vi "Set Refnums.vi"   [LabVIEW 2012]
uses:
  <vilib>/Rock Robotics/WPI/DriverStation/WPI_DriverStationRobotMode2.ctl
  Global Refnums.vi
  Robot Global Data.vi
  Global Variables.vi
types:
  T1 = typedef "WPI_DriverStationRobotMode2.ctl" = enum16{"Autonomous Disabled", "Autonomous Enabled", "Teleop Disabled", "Teleop Enabled", "Timeout", "Finish", "Test Disabled", "Test Enabled"}
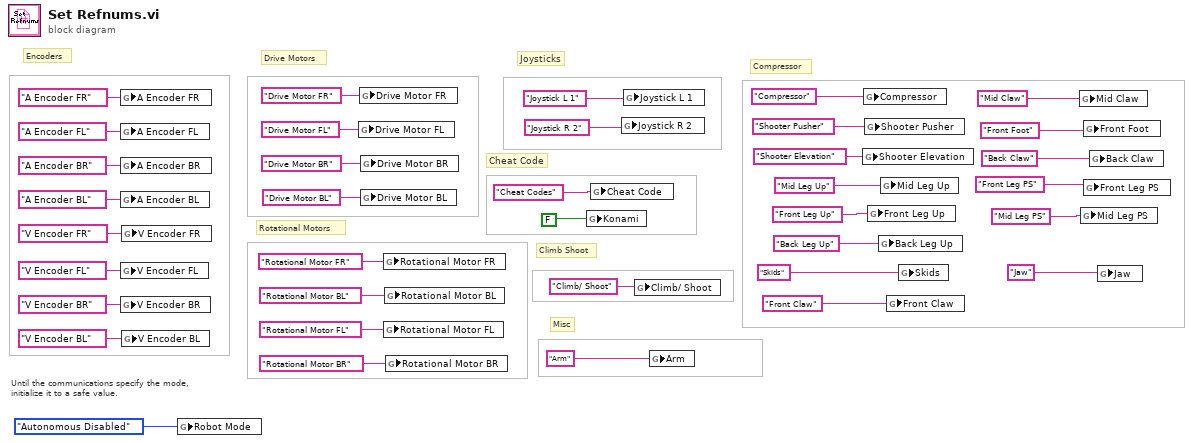
[diagram p0: block diagram]
diagram:
  # "Misc"
  # "Climb Shoot"
  # "Cheat Code"
  # "Until the communications specify the mode,\ninitialize it to a safe value."
  # "Compressor"
  # "Joysticks"
  # "Rotational Motors"
  # "Encoders"
  # "Drive Motors"
  n1 = global write "Global Refnums.vi" "A Encoder FR"("A Encoder FR") -> ()
  n2 = global write "Global Refnums.vi" "A Encoder FL"("A Encoder FL") -> ()
  n3 = global write "Global Refnums.vi" "A Encoder BR"("A Encoder BR") -> ()
  n4 = global write "Global Refnums.vi" "A Encoder BL"("A Encoder BL") -> ()
  n5 = global write "Global Refnums.vi" "V Encoder FL"("V Encoder FL") -> ()
  n6 = global write "Global Refnums.vi" "V Encoder BR"("V Encoder BR") -> ()
  n7 = global write "Global Refnums.vi" "V Encoder FR"("V Encoder FR") -> ()
  n8 = global write "Global Refnums.vi" "V Encoder BL"("V Encoder BL") -> ()
  n9 = global write "Robot Global Data.vi" "Robot Mode"(WPI_DriverStationRobotMode2."Autonomous Disabled" ("Robot Mode")) -> ()
  n10 = global write "Global Refnums.vi" "Drive Motor FL"("Drive Motor FL") -> ()
  n11 = global write "Global Refnums.vi" "Drive Motor FR"("Drive Motor FR") -> ()
  n12 = global write "Global Refnums.vi" "Drive Motor BR"("Drive Motor BR") -> ()
  n13 = global write "Global Refnums.vi" "Drive Motor BL"("Drive Motor BL") -> ()
  n14 = global write "Global Refnums.vi" "Rotational Motor FR"("Rotational Motor FR") -> ()
  n15 = global write "Global Refnums.vi" "Rotational Motor FL"("Rotational Motor FL") -> ()
  n16 = global write "Global Refnums.vi" "Rotational Motor BL"("Rotational Motor BL") -> ()
  n17 = global write "Global Refnums.vi" "Rotational Motor BR"("Rotational Motor BR") -> ()
  n18 = global write "Global Variables.vi" "Konami"(FALSE) -> ()
  n19 = global write "Global Refnums.vi" "Cheat Code"("Cheat Codes" ("refnum name")) -> ()
  n20 = global write "Global Refnums.vi" "Joystick R 2"("Joystick R 2") -> ()
  n21 = global write "Global Refnums.vi" "Joystick L 1"("Joystick L 1") -> ()
  n22 = global write "Global Refnums.vi" "Climb/ Shoot"("Climb/ Shoot") -> ()
  n23 = global write "Global Refnums.vi" "Arm"("Arm" ("Arm")) -> ()
  n24 = global write "Global Refnums.vi" "Shooter Elevation"("Shooter Elevation" ("refnum name")) -> ()
  n25 = global write "Global Refnums.vi" "Compressor"("Compressor" ("refnum name")) -> ()
  n26 = global write "Global Refnums.vi" "Shooter Pusher"("Shooter Pusher" ("refnum name")) -> ()
  n27 = global write "Global Refnums.vi" "Front Leg Up"("Front Leg Up" ("refnum name")) -> ()
  n28 = global write "Global Refnums.vi" "Back Leg Up"("Back Leg Up" ("refnum name")) -> ()
  n29 = global write "Global Refnums.vi" "Mid Leg Up"("Mid Leg Up" ("refnum name")) -> ()
  n30 = global write "Global Refnums.vi" "Front Claw"("Front Claw" ("refnum name")) -> ()
  n31 = global write "Global Refnums.vi" "Skids"("Skids" ("refnum name")) -> ()
  n32 = global write "Global Refnums.vi" "Mid Claw"("Mid Claw" ("refnum name")) -> ()
  n33 = global write "Global Refnums.vi" "Mid Leg PS"("Mid Leg PS" ("refnum name")) -> ()
  n34 = global write "Global Refnums.vi" "Front Foot"("Front Foot" ("refnum name")) -> ()
  n35 = global write "Global Refnums.vi" "Front Leg PS"("Front Leg PS" ("refnum name")) -> ()
  n36 = global write "Global Refnums.vi" "Back Claw"("Back Claw" ("refnum name")) -> ()
  n37 = global write "Global Refnums.vi" "Jaw"("Jaw") -> ()
